vi "Configure Modbus TCP Server.vi"(8 "error in (no error)":errorcluster, 9 "Modbus TCP server configuration":T1 {"protocol" items=["RTU", "ASCII", "TCP"]}, 10 "server index":u16, 11 "PLBB in":refnum<class "PL BlackBox Modbus Client.lvclass">) -> (0 "error out":errorcluster, 3 "PLBB out":refnum<class "PL BlackBox Modbus Client.lvclass">)   [LabVIEW 2015, in "PL BlackBox Modbus Client.lvclass"]
doc: "Configures the Modbus TCP server."
uses:
  PL BlackBox Modbus Client.lvclass
  <vilib>/plasmapper/PL Modbus Client/PL Modbus Client.lvclass
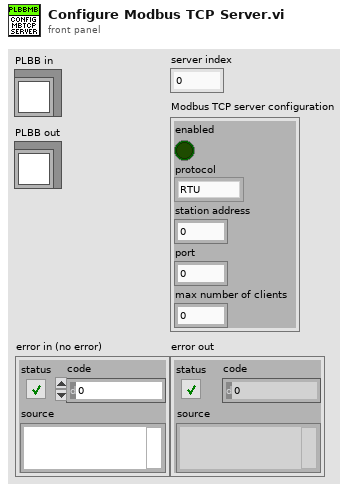
[diagram p1: front panel]
types:
  T1 = cluster{"enabled":bool, "protocol":u16, "station address":u16, "port":u16, "max number of clients":u16}
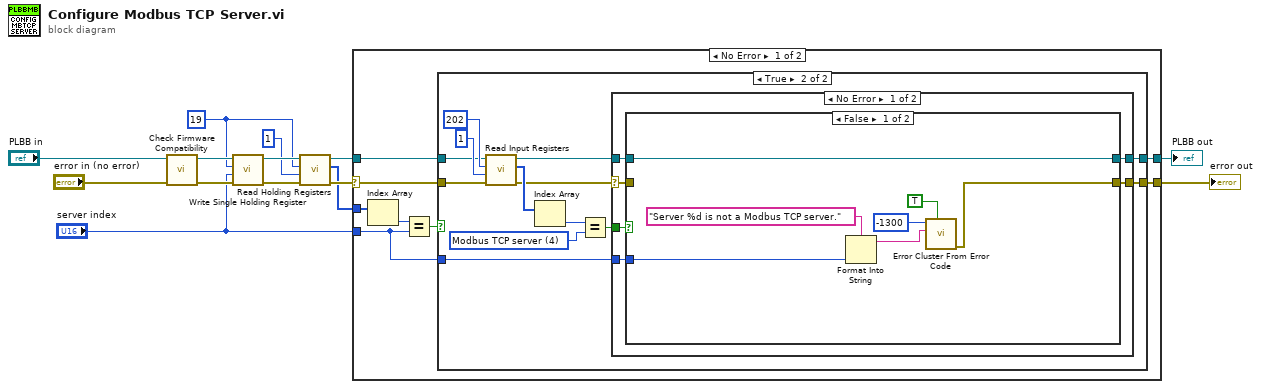
[diagram p0: block diagram]
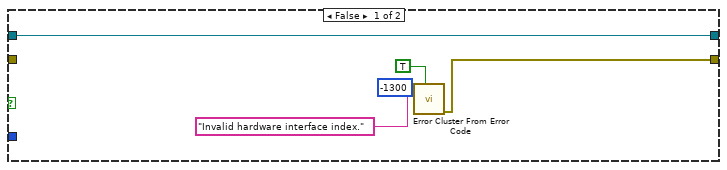
[diagram p2: hidden frame]
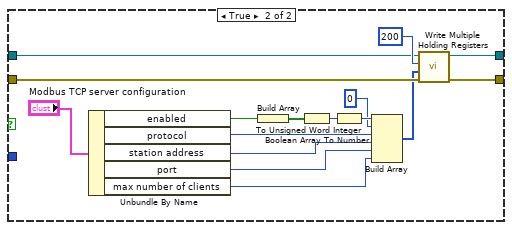
[diagram p3: hidden frame]
diagram:
  w6 = u16 19 ("address")
  n1 = call-dynamic "Check Firmware Compatibility.vi"("error in (no error)"="error in (no error)", "PLBB in"="PLBB in") -> ("error out"=w9:errorcluster, "PLBB out"=w10:refnum<class "PL BlackBox Modbus Client.lvclass">)  [unwired: 8 in]
  n2 = call <vilib>:"Write Single Holding Register.vi"("error in (no error)"=w9, "value"="server index", "address"=w6, "MODBUS in"=w10) -> ("error out"=w5:errorcluster, "MODBUS out"=w8:refnum<class "PL BlackBox Modbus Client.lvclass">)  [unwired: 6 in]
  n3 = call <vilib>:"Read Holding Registers.vi"("error in (no error)"=w5, "number of holding registers"=u16 1 ("address"), "address"=w6, "MODBUS in"=w8) -> ("error out"=w4:errorcluster, "values"=w2:u16[], "MODBUS out"=w3:refnum<class "PL BlackBox Modbus Client.lvclass">)  [unwired: 5 in]
  n4 = case shown="No Error" w4 {
    selector: w4 -> [w16 w72]
    tunnel: [w22 w72] -> w14
    tunnel: [w21 w73] -> w13
    tunnel: w3 -> [w17 w73]
    tunnel: w2 -> [w20 _]
    tunnel: "server index" -> [w15 _]
    frame No Error {
      n5 = Index Array(array=w20) -> (element=w19:u16)  [unwired: 1 in]
      n6 = Equal?(x=w19, y=w15) -> (x = y?=w18:bool)
      n7 = case shown="True" w18 {
        tunnel: [w23 w30] -> w22
        tunnel: [w27 w31] -> w21
        tunnel: w17 -> [w27 w38]
        tunnel: w16 -> [_ w37]
        tunnel: w15 -> [_ w29]
        frame False {
          n8 = call <vilib>:"Error Cluster From Error Code.vi"("show call chain? (False)"=TRUE, "error message (\"\")"="Invalid hardware interface index." ("error message (\"\")"), "error code (0)"=-1300) -> ("error out"=w23:errorcluster)  [unwired: 6 in]
        }
        frame True {
          w28 = u16 4 items=["Unknown", "UART server", "Network server", "Modbus serial server", "Modbus TCP server"] ("type")
          n9 = call <vilib>:"Read Input Registers.vi"("error in (no error)"=w37, "number of input registers"=u16 1 ("address"), "address"=u16 202, "MODBUS in"=w38) -> ("error out"=w33:errorcluster, "values"=w36:u16[], "MODBUS out"=w32:refnum<class "PL BlackBox Modbus Client.lvclass">)  [unwired: 5 in]
          n10 = Index Array(array=w36) -> (element=w35:u16)  [unwired: 1 in]
          n11 = Equal?(x=w35, y=w28) -> (x = y?=w34:bool)
          n12 = case shown="No Error" w33 {
            selector: w33 -> [w44 w70]
            tunnel: w34 -> [w46 _]
            tunnel: [w41 w71] -> w31
            tunnel: w32 -> [w45 w71]
            tunnel: [w42 w70] -> w30
            tunnel: w29 -> [w43 _]
            frame No Error {
              n13 = case shown="False" w46 {
                tunnel: w45 -> [w47 w65]
                tunnel: w44 -> [_ w64]
                tunnel: w43 -> [w50 _]
                tunnel: [w48 w68] -> w42
                tunnel: [w47 w69] -> w41
                frame False {
                  n14 = Format Into String(format string="Server %d is not a Modbus TCP server." ("error message (\"\")"), w50) -> (resulting string=w49:string)  [unwired: 2 in, 1 out]
                  n15 = call <vilib>:"Error Cluster From Error Code.vi"("show call chain? (False)"=TRUE, "error message (\"\")"=w49, "error code (0)"=-1300) -> ("error out"=w48:errorcluster)  [unwired: 6 in]
                }
                frame True {
                  n16 = Unbundle By Name("Modbus TCP server configuration") -> ("enabled"=w61:bool, "protocol"=w57:u16, "station address"=w56:u16, "port"=w55:u16, "max number of clients"=w54:u16)
                  n17 = Build Array(w61) -> (w62:bool[])
                  n18 = Boolean Array To Number(Boolean array=w62) -> (number=w63:u32)
                  n19 = To Unsigned Word Integer(number=w63) -> (unsigned 16bit integer=w60:u16)
                  n20 = Build Array(w60, u16 0 ("element"), w57, w56, w55, w54) -> (w59:u16[])
                  n21 = call <vilib>:"Write Multiple Holding Registers.vi"("error in (no error)"=w64, "values"=w59, "address"=u16 200, "MODBUS in"=w65) -> ("error out"=w68:errorcluster, "MODBUS out"=w69:refnum<class "PL BlackBox Modbus Client.lvclass">)  [unwired: 6 in]
                }
              }
            }
            frame Error {
            }
          }
        }
      }
    }
    frame Error {
    }
  }
  "error out" <- w14
  "PLBB out" <- w13
